vi "Trans.vi"(1 "Y":dbl, 2 "Array 4":dbl[][](array[numeric])) -> (0 "Y value":dbl)   [LabVIEW 2020]
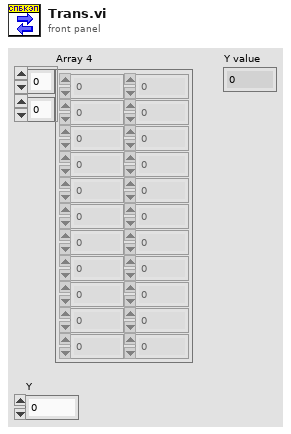
[diagram p1: front panel]
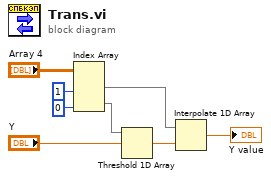
[diagram p0: block diagram]
diagram:
  n1 = Index Array(array="Array 4", index (col) #1=1 ("disabled index (col)"), index (col) #2=0 ("index (col)")) -> (element #1=w2:dbl[], element #2=w5:dbl[])  [unwired: 2 in]
  n2 = Threshold 1D Array(2:"Y", 3:w5) -> (0:w1:dbl)  [unwired: 1 in]
  n3 = Interpolate 1D Array(1:w1, 2:w2) -> (0:→"Y value":dbl)
